vi "ReadHTTPHeader.vi"(10 "Data":string="HTTP/1.1  403 Forbidden\r\nServer: websockets-LabVIEW/1.6\r\n\r\n") -> (0 "Header Found":bool, 1 "HTTP Header":string, 2 "Data Out":string="HTTP/1.1  403 Forbidden\r\nServer: websockets-LabVIEW/1.6\r\n\r\n")   [LabVIEW 2016, in "WebSocket Actors.lvlib" / "WebSocket Server.lvclass"]
doc: "WebSockets 1.6.0.22\nSam Sharp - MediaMongrels Ltd\nCopyright (c) 2016, MediaMongrels Ltd"
uses:
  WebSocket Server.lvclass
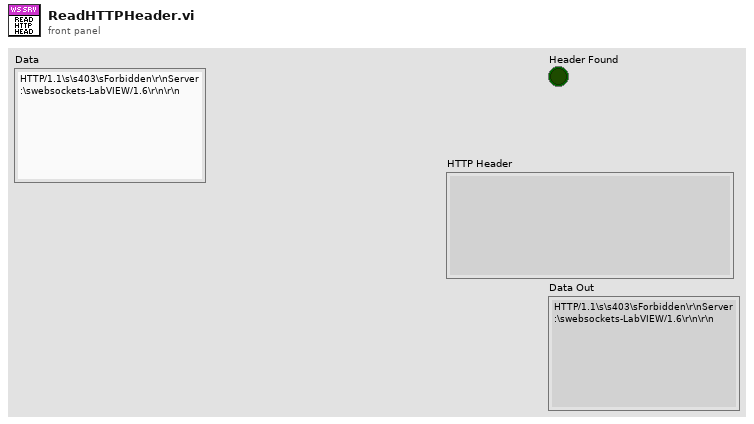
[diagram p1: front panel]
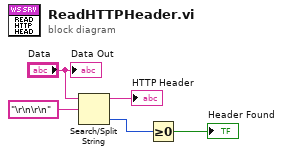
[diagram p0: block diagram]
diagram:
  n1 = Search/Split String(string="Data", search string/char (-)="\r\n\r\n") -> (substring before match=→"HTTP Header":string, offset of match=w2:i32)  [unwired: 1 in, 1 out]
  n2 = Greater Or Equal To 0?(x=w2) -> (x >= 0?=→"Header Found":bool)
  "Data Out" <- "Data"
